vi "Translation3d_Create.vi"(9 "Z":dbl, 10 "Y":dbl, 11 "X":dbl) -> (3 "TRANSLATION3D":T1 {"Z" format="%14.3f"; "Y" format="%14.3f"; "X" format="%14.3f"})   [LabVIEW 2019, in "Trajectory_Library.lvlib"]
doc: "Constructs a Translation3d with the X, Y, and Z components equal to the provided values.\n\nParameters:\n - X - The x component of the translation.\n - Y - The y component of the translation.\n - Z - The z component of the translation.\n\nReturns\n - TRANSLATION3D - The TRANSLATION3D data structure"
uses:
  Trajectory_Library.lvlib
  TRANSLATION3D.ctl
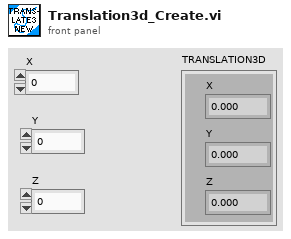
[diagram p1: front panel]
types:
  T1 = typedef "Trajectory_Library.lvlib/TRANSLATION3D.ctl" = cluster{"X":dbl, "Y":dbl, "Z":dbl}
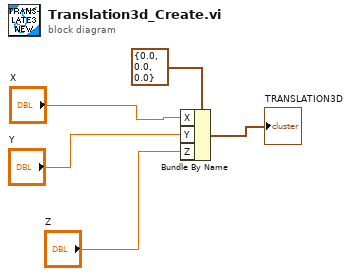
[diagram p0: block diagram]
diagram:
  n1 = Bundle By Name(cluster=T1 {"X"=0.0, "Y"=0.0, "Z"=0.0} ("TRANSLATION"), "X"="X", "Y"="Y", "Z"="Z") -> (→"TRANSLATION3D":T1)
